vi "TSC Material Tab Color Levels--constant.vi"() -> (2 "tab color levels":string[](array[string]))   [LabVIEW 2021, in "Material SubVIs.lvlib"]
doc: "CONSTANT VI defines the constant value for the tab color Levels that are shown in the right click menu and are used in color application.\n\n<b>Code Developed By:</b> +\nDaniel Coons +\nTechnology Service Corporation +\nwww.tsc.com/atcs"
uses:
  Material SubVIs.lvlib
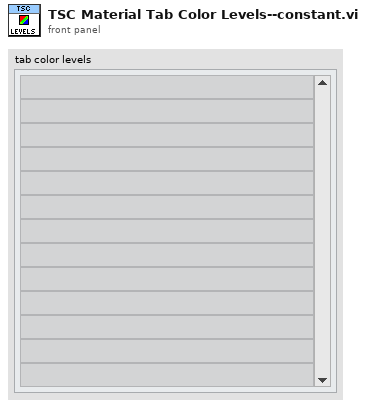
[diagram p1: front panel]
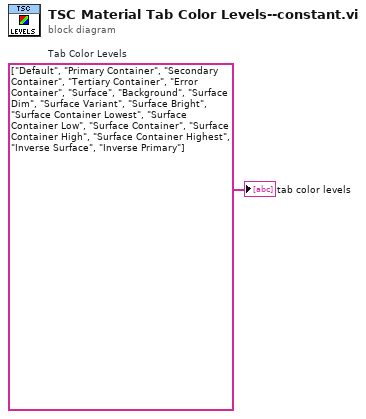
[diagram p0: block diagram]
diagram:
  w1 = string[] ["Default", "Primary Container", "Secondary Container", "Tertiary Container", "Error Container", "Surface", "Background", "Surface Dim", "Surface Variant", "Surface Bright", "Surface Container Lowest", "Surface Container Low", "Surface Container", "Surface Container High", "Surface Container Highest", "Inverse Surface", "Inverse Primary"]  # Tab Color Levels
  "tab color levels" <- w1
